vi "save_settings.vi"(8 "error in":errorcluster, 9 "Which settings to save":cluster{"Boolean":bool, "Setting":string}[](array[cluster]) caption="Choose which settings to save:", 10 "XML File Path":path, 11 "all settings":T1={"Variable Settings"={"Measurements per Iteration"=0, "Local Data Path"=path "", "Experiment description suffix for filename (no spaces please)"="", "Network Data Path"=path "", "Copy data to network"=FALSE, "Measurement Timeout (ms)"=0, "Independent Variables"=[], "Dependent Variables"=[], "Run Test Mode"=FALSE}, "HSDIO Settings"={"Enable HSDIO Pulses"=TRUE, "Resource Name"="PXI1Slot6", "Clock Rate"=20000000.0, "Array of Script Triggers"=[], "Channels Control"=[["Hex 3D MOT b0", "1", "0", "", "", "", "", "", "", "", "", "", "", "", "", "", "", "", "", ""], ["Hex 3D MOT b0", "1", "0", "", "", "", "", "", "", "", "", "", "", "", "", "", "", "", "", ""], ["repumper bit0", "1", "0", "", "", "", "", "", "", "", "", "", "", "", "", "", "", "", "", ""], ["Trap Array beam switch", "1", "0", "", "", "", "", "", "", "", "", "", "", "", "", "", "", "", "", ""], ["2D MOT switch", "1", "0", "", "", "", "", "", "", "", "", "", "", "", "", "", "", "", "", ""], ["Hamamatsu CCD trigger", "1", "0", "", "", "", "", "", "", "", "", "", "", "", "", "", "", "", "", ""], ["Luca CCD trigger", "1", "0", "", "", "", "", "", "", "", "", "", "", "", "", "", "", "", "", ""], ["broken", "", "", "", "", "", "", "", "", "", "", "", "", "", "", "", "", "", "", ""], ["repumper bit1", "1", "0", "", "", "", "", "", "", "", "", "", "", "", "", "", "", "", "", ""], ["blow away", "1", "0", "", "", "", "", "", "", "", "", "", "", "", "", "", "", "", "", ""], ["trap shutter", "1", "0", "", "", "", "", "", "", "", "", "", "", "", "", "", "", "", "", ""], ["1038 switch", "1", "0", "", "", "", "", "", "", "", "", "", "", "", "", "", "", "", "", ""], ["", "", "", "", "", "", "", "", "", "", "", "", "", "", "", "", "", "", "", ""], ["", "", "", "", "", "", "", "", "", "", "", "", "", "", "", "", "", "", "", ""], ["", "", "", "", "", "", "", "", "", "", "", "", "", "", "", "", "", "", "", ""], ["", "", "", "", "", "", "", "", "", "", "", "", "", "", "", "", "", "", "", ""], ["", "", "", "", "", "", "", "", "", "", "", "", "", "", "", "", "", "", "", ""], ["", "", "", "", "", "", "", "", "", "", "", "", "", "", "", "", "", "", "", ""], ["", "", "", "", "", "", "", "", "", "", "", "", "", "", "", "", "", "", "", ""], ["", "", "", "", "", "", "", "", "", "", "", "", "", "", "", "", "", "", "", ""], ["", "", "", "", "", "", "", "", "", "", "", "", "", "", "", "", "", "", "", ""], ["", "", "", "", "", "", "", "", "", "", "", "", "", "", "", "", "", "", "", ""], ["", "", "", "", "", "", "", "", "", "", "", "", "", "", "", "", "", "", "", ""], ["", "", "", "", "", "", "", "", "", "", "", "", "", "", "", "", "", "", "", ""], ["", "", "", "", "", "", "", "", "", "", "", "", "", "", "", "", "", "", "", ""], ["", "", "", "", "", "", "", "", "", "", "", "", "", "", "", "", "", "", "", ""], ["", "", "", "", "", "", "", "", "", "", "", "", "", "", "", "", "", "", "", ""], ["", "", "", "", "", "", "", "", "", "", "", "", "", "", "", "", "", "", "", ""], ["", "", "", "", "", "", "", "", "", "", "", "", "", "", "", "", "", "", "", ""], ["", "", "", "", "", "", "", "", "", "", "", "", "", "", "", "", "", "", "", ""], ["", "", "", "", "", "", "", "", "", "", "", "", "", "", "", "", "", "", "", ""]], "Pulse Generation Script"="script script1\n     Generate RedTrap_compress_temp\nend script", "Start Trigger"={"Wait for start trigger?"=FALSE, "source (PFI 0)"="PFI0", "edge (rising)"=12}, "Hardware alignment quantum\n(in samples)"=1, "Inital State"="", "Idle State"="", "Active Channels"="", "Array of Waveforms"=[]}, "DAQmx Pulse Settings"={"Enable DAQmx Pulses"=FALSE, "DAQmx Physical Channels"="", "Clock Rate"=0.0, "units/sec (ms=1000)"=0.0, "Start Trigger"={"Wait for start trigger?"=FALSE, "source"="", "edge"=0}, "Timing Sequence Control"=[]}, "DDS Settings"={"Enable DDS"=FALSE, "Array of DDS Boxes"=[]}, "Camera settings"={"Analog Gain (0-5)"=4, "Exposure Time"=0.01, "EM Gain (0-255)"=0, "Trigger Polarity"="ATP P", "External Trigger Mode"="EMD E", "Scan Speed"="SSP H", "External Trigger Source"="ESC B", "Scan Mode"="SMD N", "Super Pixel Binning\n(if enabled in Scan Mode)"="SPX 1", "Camera Sub-array acquisition region\n(if enabled in scan mode)"={"Left"=0, "Top"=0, "Width"=0, "Height"=0}, "Use camera?"=FALSE, "# image buffers"=100, "shots per measurement"=100, "Force images to U16"=FALSE, "Low Light Sensitivity"="LLS 0", "cooling"="CSW F", "fan"="FAN F", "Frame Grabber acquisition region"={"Left"=0, "Top"=0, "Right"=0, "Bottom"=0}}, "Counter Settings"={"Enable Counters"=FALSE, "Array of Counter Settings"=[]}, "Filter Cluster"={"Counter Filter thresholds"=[], "Data Filters\nROI Minimum Thresholds"=[]}, "Analog Output Parameters"={"Enable Analog Out?"=FALSE, "Physical Channel"="PXI1Slot2/ao0:2", "Minimum Value"=-10.0, "Maximum Value"=10.0, "Samples per second"=0.0, "Total AO Time (seconds)"=0.0, "Start Trigger"={"Wait for start trigger?"=FALSE, "source"="/Dev1/PFI0", "edge"=10280}, "Analog Output Waveforms (channel, time)"=[]}, "Notes"="", "HP83623A Generator Settings Array"=[], "Iteration Graph Settings"={"Plot Regions"="", "Plot Shots"=""}, "PI Piezo Settings"={"Enable"=FALSE, "Array of Piezo Controllers"=[]}, "Andor settings"={"Andor Path"=path "", "Copy any Andor files"=FALSE, "Wait time before copying Andor files (ms)"=0}, "Measurement Chart Settings"={"Which regions to plot (comma separated)"="", "Which shot to plot"=0}, "HP8662A Synthesized Signal Generator Array"=[], "HP83712B Synthesized CW Generator Array"=[], "TTL input"={"Enable"=FALSE, "lines"=""}} {"Variable Settings"."Independent Variables"."# steps" min=1 step=1; "Variable Settings"."Measurements per Iteration" min=1 step=1; "HSDIO Settings"."Hardware alignment quantum\n(in samples)" min=1 step=1; "HSDIO Settings"."Array of Script Triggers"."level" items=["High Level"=34, "Low Level"=35]; "HSDIO Settings"."Array of Script Triggers"."edge" items=["Rising Edge"=12, "Falling Edge"=13]; "HSDIO Settings"."Start Trigger"."edge (rising)" items=["Rising Edge"=12, "Falling Edge"=13]; "HSDIO Settings"."Clock Rate" min=0.0 max=200000000.0 format="%.2p"; "DAQmx Pulse Settings"."Start Trigger"."edge" items=["Rising"=10280, "Falling"=10171]; "DAQmx Pulse Settings"."Clock Rate" min=0.0 max=200000000.0 format="%.2p"; "Camera settings"."Frame Grabber acquisition region"."Bottom" max=512 step=1; "Camera settings"."Frame Grabber acquisition region"."Right" max=512 step=1; "Camera settings"."Frame Grabber acquisition region"."Top" max=512 step=1; "Camera settings"."Frame Grabber acquisition region"."Left" max=512 step=1; "Camera settings"."shots per measurement" min=0 step=1; "Camera settings"."# image buffers" min=0 step=1; "Camera settings"."Camera Sub-array acquisition region\n(if enabled in scan mode)"."Height" min=16 max=512 step=16; "Camera settings"."Camera Sub-array acquisition region\n(if enabled in scan mode)"."Width" min=16 max=512 step=16; "Camera settings"."Camera Sub-array acquisition region\n(if enabled in scan mode)"."Top" max=496 step=16; "Camera settings"."Camera Sub-array acquisition region\n(if enabled in scan mode)"."Left" max=496 step=16; "Camera settings"."Analog Gain (0-5)" max=5 step=1; "Counter Settings"."Array of Counter Settings"."Binwidth (ms)" format="%0.2f"; "Analog Output Parameters"."Start Trigger"."edge" items=["Rising"=10280, "Falling"=10171]; "Analog Output Parameters"."Maximum Value" format="%0.2f"; "Analog Output Parameters"."Minimum Value" format="%0.2f"}) -> (0 "error out":errorcluster)   [LabVIEW 2013]
uses:
  ExperimentVariables/ExperimentVariables.lvclass
  HSDIO/HSDIO.lvclass
  DAQmx_pulse_out/DAQmx_pulse_out.lvclass
  DDS/DDS.lvclass
  Camera/Hamamatsu_C9100-13/Hamamatsu_C9100-13.lvclass
  Counter/Counter.lvclass
  Analog_output/Analog_Output.lvclass
  GPIB/GPIB.lvclass
  PI_piezo/PI_Piezo.lvclass
  Analog_output/AO_settings.ctl
  filters/filters.ctl
  Counter/Counter_Settings_Control.ctl
  Camera/Hamamatsu_C9100-13/camera_setup.ctl
  <vilib>/ni845x/ni845x.llb/ni845xControl.ctl
  DDS drivers v3/DDS_box_device_reference.ctl
  DDS drivers v3/DDS RAM mode.ctl
  DDS drivers v3/DDS_box_cluster.ctl
  DDS drivers v3/Array_of_DDS_Boxes.ctl
  DDS/DDS_Settings_Cluster.ctl
  DAQmx_pulse_out/settings.ctl
  <instrlib>/niHSDIO/niHSDIO.llb/niHSDIO_ctl Trigger Source Values (Ring).ctl
  <instrlib>/niHSDIO/niHSDIO.llb/niHSDIO_ctl Trigger DigEdge - Edge Values (Ring).ctl
  <instrlib>/niHSDIO/niHSDIO.llb/niHSDIO_ctl Trigger Script - trigID Values (Ring).ctl
  <instrlib>/niHSDIO/niHSDIO.llb/niHSDIO_ctl Trigger DigLvl - Level Values (Ring).ctl
  HSDIO/HSDIO_settings.ctl
  ExperimentVariables/Variable_Settings.ctl
  all_settings.ctl
  GPIB/HP83623A_RF_Generator/HP83623A_array.ctl
  GPIB/HP83623A_RF_Generator/HP83623A_RF_Generator.lvclass
  PI_piezo/settings.ctl
  Camera/Andor/Andor_settings.ctl
  gui/measurement_graph.ctl
  GPIB/RF_Generator_settings.ctl
  GPIB/RF_Generator_settings_array.ctl
  DDS drivers v3/DDS_profile.ctl
  DDS drivers v3/DDS_channel.ctl
  DDS drivers v3/array_of_DDS_profiles.ctl
  DDS drivers v3/array_of_DDS_channels.ctl
  TTL_input/TTL_input_settings.ctl
  TTL_input/TTL_input.lvclass
  HSDIO/waveform.ctl
  PI_piezo/piezo_channel.ctl
  PI_piezo/piezo_controller.ctl
  GPIB/HP83623A_RF_Generator/HP83623A.ctl
panel:
  out "concatenated string":string
  # "Parameters will be evaluated once at the beginning of the experiment from top to bottom, \nso any parameter may depend on all those above it.\nVariables will be evaluated each iteration.\nParameters and Variables may be used in various other experiment settings, as noted.\nSee LabView Help -> Formula Node and Expression Node Functions for a list of available functions."
  # "Regions of Interest -->"
  # "Shots\n   |\n  V"
  # "Counters -->"
  # "Counter\n    bins\n       |\n      V"
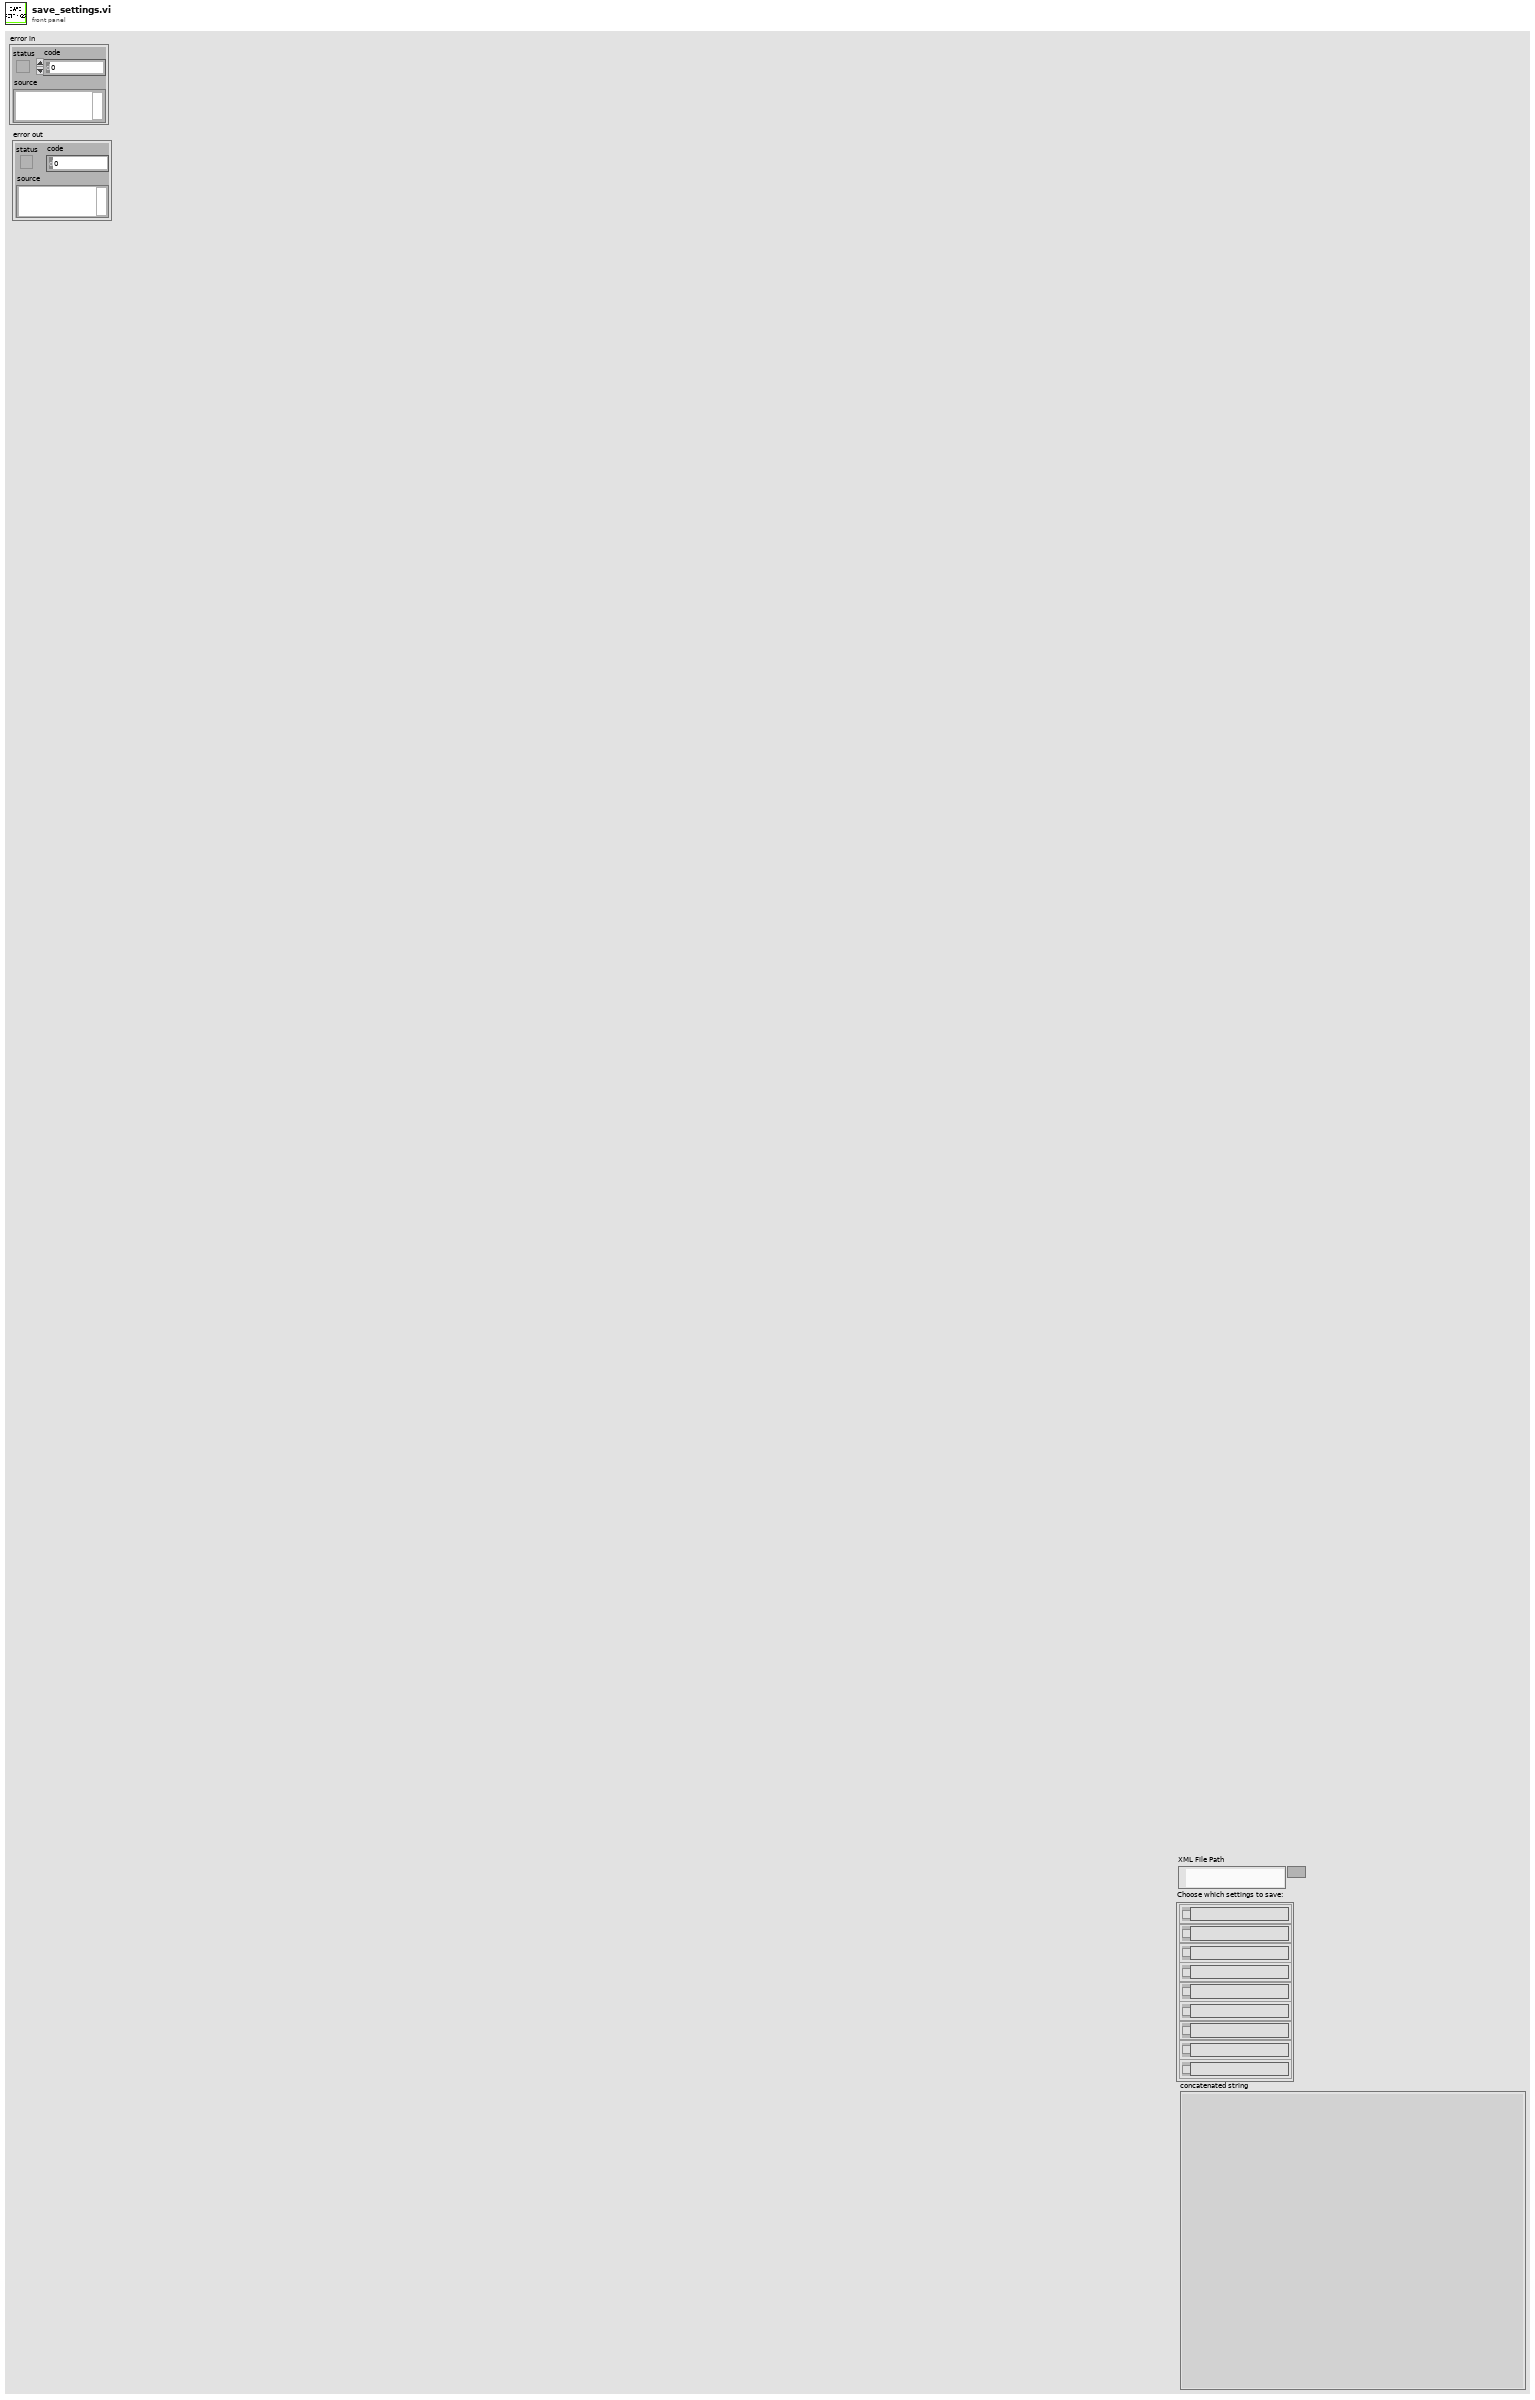
[diagram p1: front panel]
types:
  T1 = typedef "all_settings.ctl" = cluster{"Variable Settings":T2, "HSDIO Settings":T3, "DAQmx Pulse Settings":T9, "DDS Settings":T10, "Camera settings":T20, "Counter Settings":T21, "Filter Cluster":T22, "Analog Output Parameters":T23, "Notes":string, "HP83623A Generator Settings Array":T24, "Iteration Graph Settings":cluster{"Plot Regions":string, "Plot Shots":string}, "PI Piezo Settings":T26, "Andor settings":T29, "Measurement Chart Settings":T30, "HP8662A Synthesized Signal Generator Array":T31, "HP83712B Synthesized CW Generator Array":T31, "TTL input":T33}
  T2 = typedef "ExperimentVariables.lvclass/Variable_Settings.ctl" = cluster{"Measurements per Iteration":i32, "Local Data Path":path, "Experiment description suffix for filename (no spaces please)":string, "Network Data Path":path, "Copy data to network":bool, "Measurement Timeout (ms)":u32, "Independent Variables":cluster{"Description":string, "Name (a,a0...a9)":string, "min":dbl, "max":dbl, "# steps":u32}[], "Dependent Variables":cluster{"Description":string, "Name (a,a0...a9)":string, "Equation":string, "Result":dbl}[], "Run Test Mode":bool}
  T3 = typedef "HSDIO.lvclass/HSDIO_settings.ctl" = cluster{"Enable HSDIO Pulses":bool, "Resource Name":refnum<k15>, "Clock Rate":dbl, "Array of Script Triggers":cluster{"trigger id (script trigger 0)":T4, "source (PFI 0)":T5, "Trigger Type":enum32{"Edge", "Level"}, "edge":T6, "level":T7}[], "Channels Control":string[][], "Pulse Generation Script":string, "Start Trigger":cluster{"Wait for start trigger?":bool, "source (PFI 0)":T5, "edge (rising)":T6}, "Hardware alignment quantum\n(in samples)":u16, "Inital State":string, "Idle State":string, "Active Channels":string, "Array of Waveforms":T8[]}
  T4 = typedef "niHSDIO_ctl Trigger Script - trigID Values (Ring).ctl" = string
  T5 = typedef "niHSDIO_ctl Trigger Source Values (Ring).ctl" = string
  T6 = typedef "niHSDIO_ctl Trigger DigEdge - Edge Values (Ring).ctl" = i32
  T7 = typedef "niHSDIO_ctl Trigger DigLvl - Level Values (Ring).ctl" = i32
  T8 = typedef "HSDIO.lvclass/waveform.ctl" = cluster{"name":string, "transitions":u32[], "states":u8[][]}
  T9 = typedef "DAQmx_pulse_out.lvclass/settings.ctl" = cluster{"Enable DAQmx Pulses":bool, "DAQmx Physical Channels":tag, "Clock Rate":dbl, "units/sec (ms=1000)":dbl, "Start Trigger":cluster{"Wait for start trigger?":bool, "source":tag, "edge":i32}, "Timing Sequence Control":string[][]}
  T10 = typedef "DDS_Settings_Cluster.ctl" = cluster{"Enable DDS":bool, "Array of DDS Boxes":T11}
  T11 = typedef "Array_of_DDS_Boxes.ctl" = T12[]
  T12 = typedef "DDS_box_cluster.ctl" = cluster{"DDS box device reference":T13, "Array of DDS Channels (4)":T15, "Enable":bool, "Description":string}
  T13 = typedef "DDS_box_device_reference.ctl" = cluster{"NI USB-8451 device reference":T14, "DIO port":u8, "Serial Clock Rate [kHz]":u16}
  T14 = typedef "ni845xControl.ctl" = refnum<k21>
  T15 = typedef "DDS.lvclass/array_of_DDS_channels.ctl" = T16[]
  T16 = typedef "DDS.lvclass/DDS_channel.ctl" = cluster{"Power":bool, "Channel Parameters":cluster{"Ref Clock Rate [kHz]":dbl, "Full Scale Output\nPower [dBm]":dbl}, "RAM Enable":bool, "RAM Dest Type":u8, "RAM Default":cluster{"Frequency [MHz]":dbl, "Amplitude [dBm]":dbl, "Phase Offset [rad]":dbl}, "Array of DDS Profiles (8)":T17, "Description":string}
  T17 = typedef "DDS.lvclass/array_of_DDS_profiles.ctl" = T18[]
  T18 = typedef "DDS_profile.ctl" = cluster{"Single Tone":cluster{"Frequency [MHz]":dbl, "Amplitude [dBm]":dbl, "Phase Offset [rad]":dbl}, "RAM Mode ":T19, "Zero-crossing":bool, "No Dwell High":bool, "Function/Static":bool, "RAM Function Settings":string[], "RAM Static Array":dbl[], "Description":string}
  T19 = typedef "DDS RAM mode.ctl" = enum16{"Direct Switch", "Ramp Up", "Bidirectional Ramp", "Continuous Bidirectional Ramp", "Continuous Recirculate", "Direct Switch 2", "Direct Switch 3", "Direct Switch 4"}
  T20 = typedef "Hamamatsu_C9100-13.lvclass/camera_setup.ctl" = cluster{"Analog Gain (0-5)":u8, "Exposure Time":dbl, "EM Gain (0-255)":u8, "Trigger Polarity":string, "External Trigger Mode":string, "Scan Speed":string, "External Trigger Source":string, "Scan Mode":string, "Super Pixel Binning\n(if enabled in Scan Mode)":string, "Camera Sub-array acquisition region\n(if enabled in scan mode)":cluster{"Left":u16, "Top":u16, "Width":u16, "Height":u16}, "Use camera?":bool, "# image buffers":i32, "shots per measurement":i32, "Force images to U16":bool, "Low Light Sensitivity":string, "cooling":string, "fan":string, "Frame Grabber acquisition region":cluster{"Left":i32, "Top":i32, "Right":i32, "Bottom":i32}}
  T21 = typedef "Counter.lvclass/Counter_Settings_Control.ctl" = cluster{"Enable Counters":bool, "Array of Counter Settings":cluster{"Counter Channel":tag, "Time-Bin Clock Channel":tag, "Binwidth (ms)":dbl}[]}
  T22 = typedef "filters.ctl" = cluster{"Counter Filter thresholds":u32[][], "Data Filters\nROI Minimum Thresholds":u64[][]}
  T23 = typedef "Analog_Output.lvclass/AO_settings.ctl" = cluster{"Enable Analog Out?":bool, "Physical Channel":tag, "Minimum Value":dbl, "Maximum Value":dbl, "Samples per second":dbl, "Total AO Time (seconds)":dbl, "Start Trigger":cluster{"Wait for start trigger?":bool, "source":tag, "edge":i32}, "Analog Output Waveforms (channel, time)":dbl[][]}
  T24 = typedef "HP83623A_RF_Generator.lvclass/HP83623A_array.ctl" = T25[]
  T25 = typedef "HP83623A_RF_Generator.lvclass/HP83623A.ctl" = cluster{"Frequency (Hz)":dbl, "Power (dBm)":dbl, "Enabled":bool, "initialized":bool, "RF Output On/Off":bool, "External Trigger?":bool, "VISA Session":refnum<visa-resource-name>, "Generator Name":string}
  T26 = typedef "PI_Piezo.lvclass/settings.ctl" = cluster{"Enable":bool, "Array of Piezo Controllers":T27[]}
  T27 = typedef "PI_Piezo.lvclass/piezo_controller.ctl" = cluster{"Enable":bool, "Serial No.":string, "Array of Piezo Channels":T28[]}
  T28 = typedef "PI_Piezo.lvclass/piezo_channel.ctl" = cluster{"Servo":bool, "Set Position":dbl}
  T29 = typedef "Andor_settings.ctl" = cluster{"Andor Path":path, "Copy any Andor files":bool, "Wait time before copying Andor files (ms)":u16}
  T30 = typedef "measurement_graph.ctl" = cluster{"Which regions to plot (comma separated)":string, "Which shot to plot":u8}
  T31 = typedef "GPIB.lvclass/RF_Generator_settings_array.ctl" = T32[]
  T32 = typedef "GPIB.lvclass/RF_Generator_settings.ctl" = cluster{"Enable":bool, "Description":string, "GPIB channel #":u8, "Frequency (MHz)":dbl, "Power (dBm)":dbl}
  T33 = typedef "TTL_input.lvclass/TTL_input_settings.ctl" = cluster{"Enable":bool, "lines":tag}
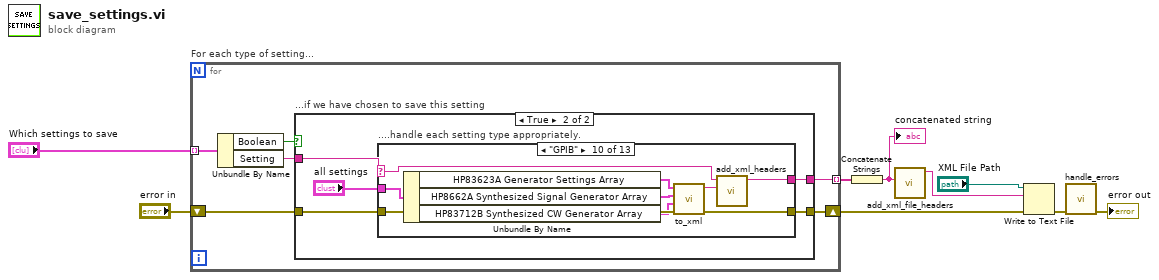
[diagram p0: block diagram]
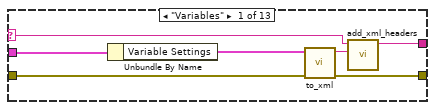
[diagram p3: hidden frame]
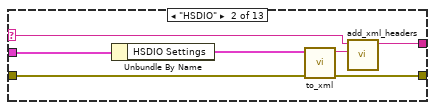
[diagram p4: hidden frame]
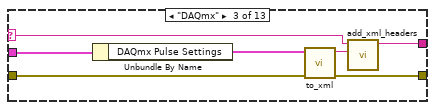
[diagram p5: hidden frame]
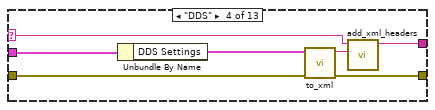
[diagram p6: hidden frame]
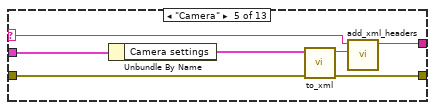
[diagram p7: hidden frame]
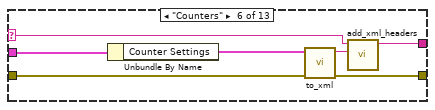
[diagram p8: hidden frame]
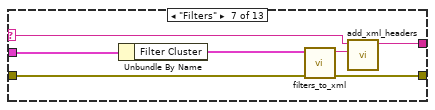
[diagram p9: hidden frame]
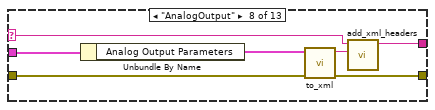
[diagram p10: hidden frame]
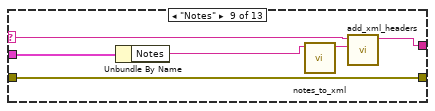
[diagram p11: hidden frame]
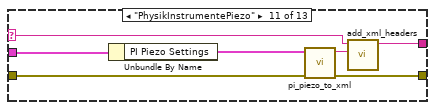
[diagram p12: hidden frame]
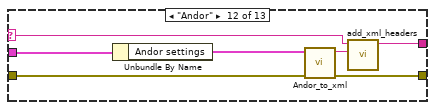
[diagram p13: hidden frame]
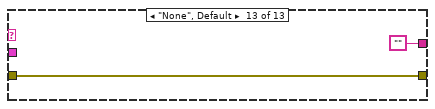
[diagram p14: hidden frame]
diagram:
  n1 = for "For each type of setting..." {
    tunnel: "Which settings to save" -> [w15] mode=indexing
    shift-right: [w12] -> w6
    shift-left: "error in" -> [w11]
    tunnel: [w10] -> w4 mode=indexing
    n2 = Unbundle By Name(w15) -> ("Boolean"=w14:bool, "Setting"=w13:string)
    n3 = case "...if we have chosen to save this setting" shown="True" w14 {
      tunnel: w13 -> [_ w19]
      tunnel: [w16 w21] -> w12
      tunnel: w11 -> [w16 w20]
      tunnel: [_ w18] -> w10
      frame False {
      }
      frame True {
        n4 = case "....handle each setting type appropriately." shown="\"GPIB\"" w19 {
          selector: w19 -> [w22 w29 w37 w43 w54 w61 w68 w75 w80 w90 w97 w105 _]
          tunnel: [w25 w32 w39 w45 w50 w58 w65 w72 w81 w87 w94 w102 w108] -> w21
          tunnel: "all settings" -> [w28 w35 w42 w49 w55 w63 w70 w77 w83 w92 w99 w106 _]
          tunnel: w20 -> [w26 w33 w40 w46 w52 w59 w66 w73 w81 w88 w95 w103 w108]
          tunnel: [w27 w34 w41 w48 w56 w62 w69 w76 w82 w91 w98 w101 ""] -> w18
          frame "Variables" {
            n5 = Unbundle By Name(w28) -> ("Variable Settings"=w24:T2)
            n6 = call "to_xml.vi"("error in"=w26, "Variable Settings"=w24) -> ("error out"=w25:errorcluster, "varible settings string"=w23:string)  [unwired: 8 in]
            n7 = call "add_xml_headers.vi"("xml"=w23, "header string"=w22) -> ("xml with headers"=w27:string)  [unwired: 9 in]
          }
          frame "HSDIO" {
            n8 = Unbundle By Name(w35) -> ("HSDIO Settings"=w31:T3)
            n9 = call "to_xml.vi"("error in"=w33, "HSDIO Settings"=w31) -> ("error out"=w32:errorcluster, "HSDIO settings string"=w30:string)  [unwired: 8 in]
            n10 = call "add_xml_headers.vi"("xml"=w30, "header string"=w29) -> ("xml with headers"=w34:string)  [unwired: 9 in]
          }
          frame "DAQmx" {
            n11 = Unbundle By Name(w42) -> ("DAQmx Pulse Settings"=w36:T9)
            n12 = call "to_xml.vi"("error in"=w40, "DAQmx Pulse Settings"=w36) -> ("error out"=w39:errorcluster, "DAQmx settings string"=w38:string)  [unwired: 8 in]
            n13 = call "add_xml_headers.vi"("xml"=w38, "header string"=w37) -> ("xml with headers"=w41:string)  [unwired: 9 in]
          }
          frame "DDS" {
            n14 = Unbundle By Name(w49) -> ("DDS Settings"=w47:T10)
            n15 = call "to_xml.vi"("error in"=w46, "DDS Settings"=w47) -> ("error out"=w45:errorcluster, "DDS settings string"=w44:string)  [unwired: 8 in]
            n16 = call "add_xml_headers.vi"("xml"=w44, "header string"=w43) -> ("xml with headers"=w48:string)  [unwired: 9 in]
          }
          frame "Camera" {
            n17 = Unbundle By Name(w55) -> ("Camera settings"=w53:T20)
            n18 = call "to_xml.vi"("error in"=w52, "Camera Setup"=w53) -> ("error out"=w50:errorcluster, "Camera Setup string"=w51:string)  [unwired: 8 in]
            n19 = call "add_xml_headers.vi"("xml"=w51, "header string"=w54) -> ("xml with headers"=w56:string)  [unwired: 9 in]
          }
          frame "Counters" {
            n20 = Unbundle By Name(w63) -> ("Counter Settings"=w60:T21)
            n21 = call "to_xml.vi"("error in"=w59, "Counter Settings"=w60) -> ("error out"=w58:errorcluster, "counter settings string"=w57:string)  [unwired: 8 in]
            n22 = call "add_xml_headers.vi"("xml"=w57, "header string"=w61) -> ("xml with headers"=w62:string)  [unwired: 9 in]
          }
          frame "Filters" {
            n23 = Unbundle By Name(w70) -> ("Filter Cluster"=w67:T22)
            n24 = call "filters_to_xml.vi"("error in"=w66, "Filter Settings"=w67) -> ("error out"=w65:errorcluster, "filter settings string"=w64:string)  [unwired: 8 in]
            n25 = call "add_xml_headers.vi"("xml"=w64, "header string"=w68) -> ("xml with headers"=w69:string)  [unwired: 9 in]
          }
          frame "AnalogOutput" {
            n26 = Unbundle By Name(w77) -> ("Analog Output Parameters"=w74:T23)
            n27 = call "to_xml.vi"("error in"=w73, "Analog Output Parameters"=w74) -> ("error out"=w72:errorcluster, "Analog Output Settings string"=w71:string)  [unwired: 8 in]
            n28 = call "add_xml_headers.vi"("xml"=w71, "header string"=w75) -> ("xml with headers"=w76:string)  [unwired: 9 in]
          }
          frame "Notes" {
            n29 = Unbundle By Name(w83) -> ("Notes"=w79:string)
            n30 = call "notes_to_xml.vi"("Notes (in)"=w79) -> ("Notes"=w78:string)  [unwired: 10 in]
            n31 = call "add_xml_headers.vi"("xml"=w78, "header string"=w80) -> ("xml with headers"=w82:string)  [unwired: 9 in]
          }
          frame "GPIB" {
            n32 = Unbundle By Name(w92) -> ("HP83623A Generator Settings Array"=w89:T24, "HP8662A Synthesized Signal Generator Array"=w85:T31, "HP83712B Synthesized CW Generator Array"=w84:T31)
            n33 = call "to_xml.vi"("error in"=w88, "HP83712B Synthesized CW Generator Array"=w84, "HP8662A Synthesized Signal Generator Array"=w85, "HP83623A Generator Settings Array"=w89) -> ("error out"=w87:errorcluster, "Spectrum Analyzer Settings string"=w86:string)  [unwired: 6 in]
            n34 = call "add_xml_headers.vi"("xml"=w86, "header string"=w90) -> ("xml with headers"=w91:string)  [unwired: 9 in]
          }
          frame "PhysikInstrumentePiezo" {
            n35 = Unbundle By Name(w99) -> ("PI Piezo Settings"=w96:T26)
            n36 = call "pi_piezo_to_xml.vi"("error in"=w95, "PI Piezo Settings"=w96) -> ("error out"=w94:errorcluster, "PI piezo settings string"=w93:string)  [unwired: 8 in]
            n37 = call "add_xml_headers.vi"("xml"=w93, "header string"=w97) -> ("xml with headers"=w98:string)  [unwired: 9 in]
          }
          frame "Andor" {
            n38 = Unbundle By Name(w106) -> ("Andor settings"=w100:T29)
            n39 = call "Andor_to_xml.vi"("error in"=w103, "Andor settings"=w100) -> ("error out"=w102:errorcluster, "settings string"=w104:string)  [unwired: 8 in]
            n40 = call "add_xml_headers.vi"("xml"=w104, "header string"=w105) -> ("xml with headers"=w101:string)  [unwired: 9 in]
          }
          frame "None", Default {
          }
        }
      }
    }
  }
  n41 = Concatenate Strings(w4) -> (w5:string)
  "concatenated string" <- w5
  n42 = call "add_xml_file_headers.vi"("xml"=w5) -> ("xml with headers"=w3:string)  [unwired: 10 in]
  n43 = Write to Text File(file (use dialog)="XML File Path", text=w3, error in=w6) -> (error out=w2:errorcluster)  [unwired: 1 in, 2 out]
  n44 = call "handle_errors.vi"("error in (no error)"=w2) -> ("error out"=→"error out":errorcluster)  [unwired: 10 in]
